vi "Main.vi"(8 "error in":errorcluster, 11 "Save Data in":refnum<class "Save Data.lvclass">) -> (0 "error out":errorcluster, 3 "Save Data out":refnum<class "Save Data.lvclass">)   [LabVIEW 2018, in "Save Data.lvclass"]
doc: "The Queued Message Handler of a Worker."
uses:
  Save Data.lvclass
  Save Data.lvclass/Save Data.ctl
  Aging View/Datas.ctl
  <vilib>/drjdpowell/SQLite Library/SQL Connection/Open (path).vi
  <vilib>/drjdpowell/SQLite Library/SQL Connection/Open (string).vi
  <vilib>/AdvancedString/Path To Command Line String.vi
  <vilib>/drjdpowell/SQLite Library/SQL Connection/Execute SQL (No results).vi
  <vilib>/drjdpowell/SQLite Library/SQL Connection/Connection.lvclass
  Initialization Data.ctl
  Aging View/Aging View.lvclass
  <vilib>/drjdpowell/SQLite Library/SQLite.lvlib
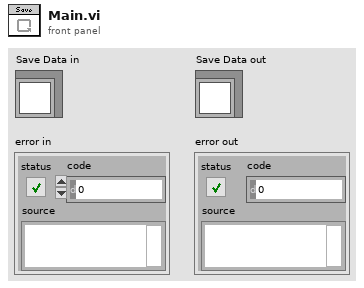
[diagram p1: front panel]
types:
  T1 = typedef "Save Data.lvclass/Initialization Data.ctl" = cluster{"MainPanel":refnum<vi>}
  T2 = typedef "Aging View.lvclass/Datas.ctl" = cluster{"Volts":dbl[], "Currents":dbl[], "Temps":dbl[]}
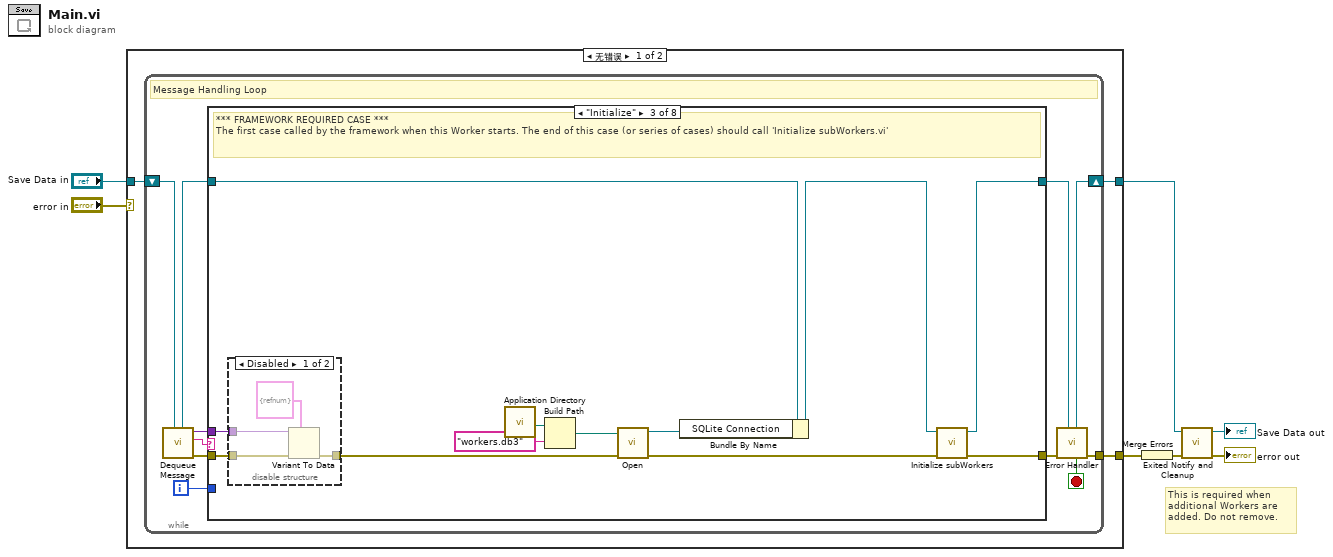
[diagram p0: block diagram]
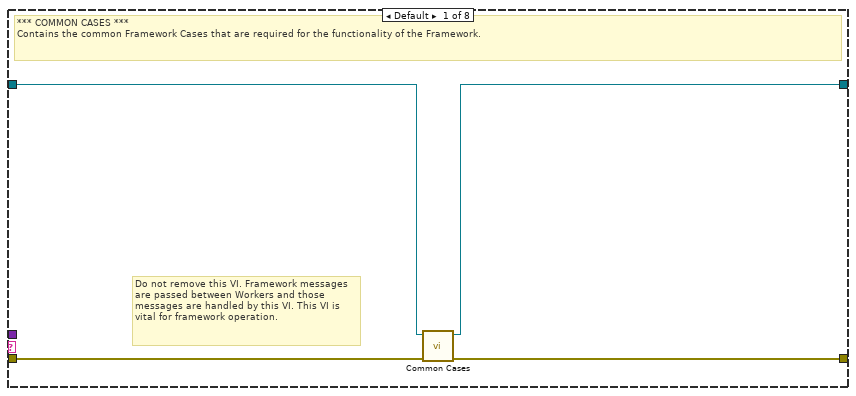
[diagram p2: hidden frame]
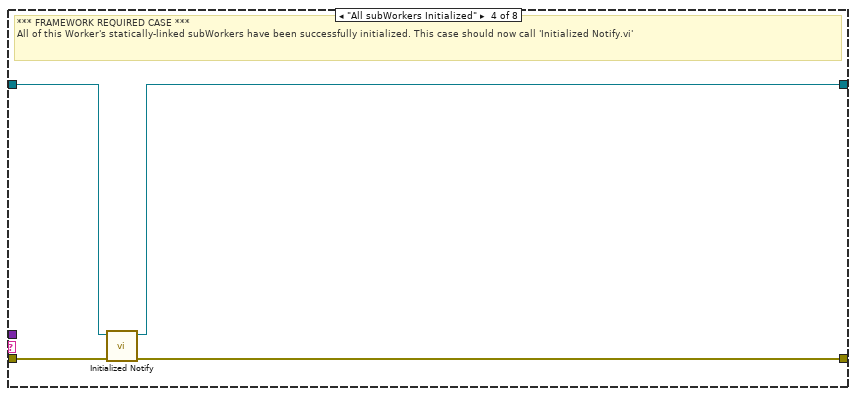
[diagram p5: hidden frame]
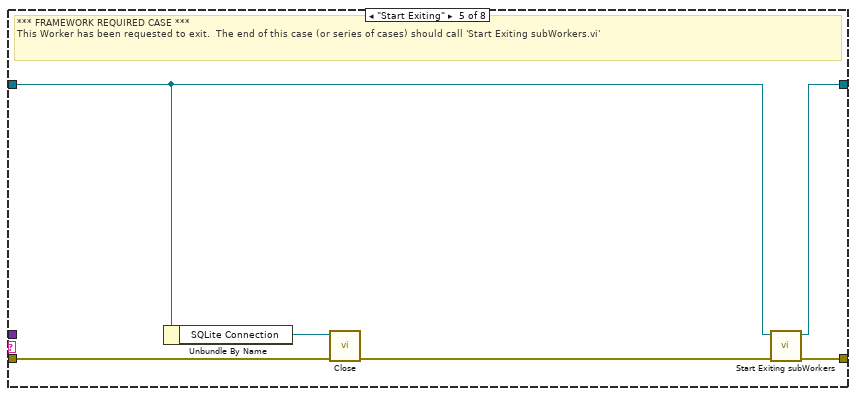
[diagram p6: hidden frame]
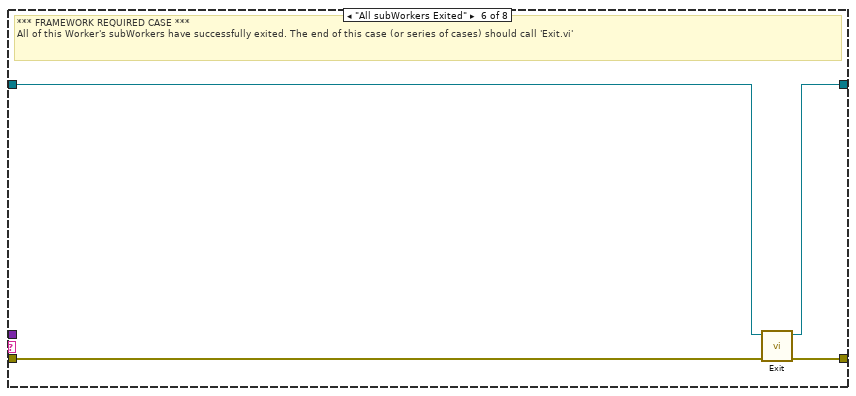
[diagram p7: hidden frame]
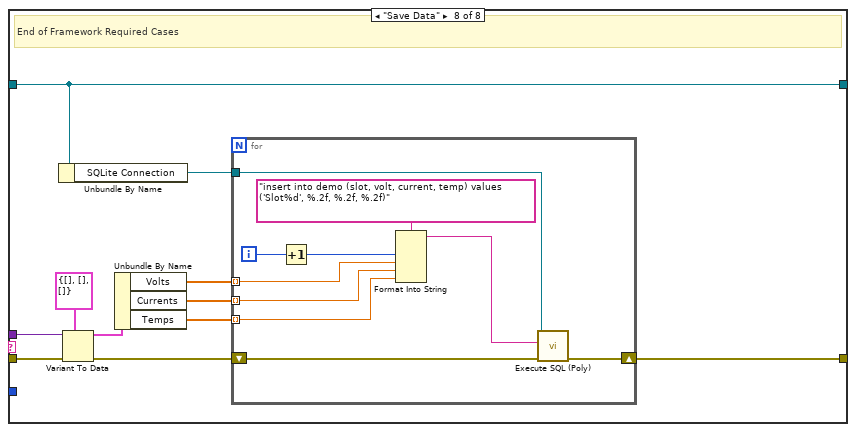
[diagram p9: hidden frame]
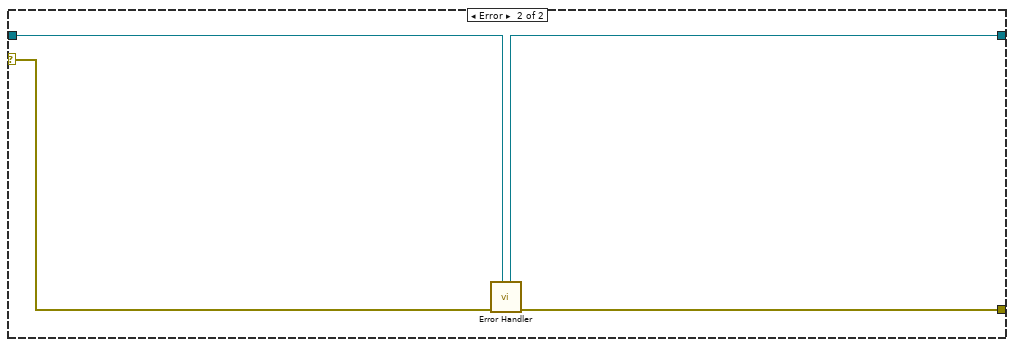
[diagram p10: hidden frame]
diagram:
  # "This is required when additional Workers are added. Do not remove."
  n1 = case shown="无错误" "error in" {
    tunnel: "Save Data in" -> [w8 w83]
    tunnel: [w10 w84] -> w6
    tunnel: [w9 w82] -> w7
    selector: "error in" -> [_ w85]
    frame No Error {
      n2 = while {
        shift-right: [w19] -> w9
        shift-left: w8 -> [w21]
        tunnel: [w20] -> w10
        i -> [w11]
        stop <- w12 stop-if-true
        # "Message Handling Loop"
        n3 = call-dynamic "Dequeue Message.vi"("Worker"=w21) -> ("error out"=w18:errorcluster, "Case out"=w13:string, "Data out"=w14:variant, "Worker out"=w16:refnum<class "Save Data.lvclass">)  [unwired: 6 in, 1 out]
        n4 = case "Worker MHL Case Structure (DO NOT CHANGE LABEL NAME)" shown="\"Initialize\"" w13 {
          tunnel: w18 -> [w25 w26 w37 w48 w52 w58 w59 w71]
          tunnel: [w24 w26 w39 w47 w54 w57 w59 w66] -> w17
          tunnel: w16 -> [w23 w27 w36 w46 w50 w56 w60 w65]
          tunnel: [w22 w27 w38 w45 w53 w55 w60 w65] -> w15
          tunnel: w14 -> [_ _ w35 _ _ _ _ w70]
          tunnel: w11 -> [_ _ _ _ _ _ _ _]
          frame Default {
            # "Do not remove this VI. Framework messages are passed between Workers and those messages are handled by this VI. This VI is vital for framework operation."
            # "*** COMMON CASES ***\nContains the common Framework Cases that are required for the functionality of the Framework."
            n5 = call-dynamic "Common Cases.vi"("error in"=w25, "Worker in"=w23) -> ("error out"=w24:errorcluster, "Worker out"=w22:refnum<class "Save Data.lvclass">)  [unwired: 8 in]
          }
          frame "------ FRAMEWORK REQUIRED CASES ------" {
            # "Start of Framework Required Cases"
          }
          frame "Initialize" {
            # "*** FRAMEWORK REQUIRED CASE ***\nThe first case called by the framework when this Worker starts. The end of this case (or series of cases) should call 'Initialize subWorkers.vi'"
            n6 = disable-structure shown="Disabled" {
              disable-tunnel: w37 -> [w43 w44]
              disable-tunnel: [w42 w44] -> w34
              disable-tunnel: w35 -> [w40 _]
              frame Disabled {
                n7 = Variant To Data(error in=w43, type=T1 {"MainPanel"=refnum} ("Cluster"), Variant=w40) -> (error out=w42:errorcluster)  [unwired: 1 out]
              }
              frame Enabled {
              }
            }
            n8 = call <vilib>:"Application Directory.vi"() -> ("Application Directory"=w33:path)
            n9 = Build Path(base path=w33, name or relative path="workers.db3") -> (appended path=w31:path)
            n10 = call-poly <vilib>:"Open.vi"("error in (no error)"=w34, "db file"=w31) -> ("error out"=w28:errorcluster, "SQLite Connection"=w29:refnum<class "Connection.lvclass">)  [unwired: 8 in]
            n11 = Bundle By Name(cluster=w36, "SQLite Connection"=w29) -> (w30:refnum<class "Save Data.lvclass">)
            n12 = call-dynamic "Initialize subWorkers.vi"("error in"=w28, "Worker"=w30) -> ("error out"=w39:errorcluster, "dup Worker out"=w38:refnum<class "Save Data.lvclass">)  [unwired: 8 in]
          }
          frame "All subWorkers Initialized" {
            # "*** FRAMEWORK REQUIRED CASE ***\nAll of this Worker's statically-linked subWorkers have been successfully initialized. This case should now call 'Initialized Notify.vi'"
            n13 = call-dynamic "Initialized Notify.vi"("error in"=w48, "Worker"=w46) -> ("error out"=w47:errorcluster, "dup Worker out"=w45:refnum<class "Save Data.lvclass">)  [unwired: 8 in]
          }
          frame "Start Exiting" {
            # "*** FRAMEWORK REQUIRED CASE ***\nThis Worker has been requested to exit.  The end of this case (or series of cases) should call 'Start Exiting subWorkers.vi'"
            n14 = Unbundle By Name(w50) -> ("SQLite Connection"=w49:refnum<class "Connection.lvclass">)
            n15 = call-dynamic "Close.vi"("error in (no error)"=w52, "SQLite Connection in"=w49) -> ("error out"=w51:errorcluster)  [unwired: 9 in]
            n16 = call-dynamic "Start Exiting subWorkers.vi"("error_in"=w51, "Worker"=w50) -> ("error out"=w54:errorcluster, "dup Worker out"=w53:refnum<class "Save Data.lvclass">)  [unwired: 8 in]
          }
          frame "All subWorkers Exited" {
            # "*** FRAMEWORK REQUIRED CASE ***\nAll of this Worker's subWorkers have successfully exited. The end of this case (or series of cases) should call 'Exit.vi'"
            n17 = call-dynamic "Exit.vi"("error_in"=w58, "Worker"=w56) -> ("error out"=w57:errorcluster, "dup Worker out"=w55:refnum<class "Save Data.lvclass">)  [unwired: 8 in]
          }
          frame "-----------------------------------------------" {
            # "End of Framework Required Cases"
          }
          frame "Save Data" {
            # "End of Framework Required Cases"
            n18 = Unbundle By Name(w65) -> ("SQLite Connection"=w64:refnum<class "Connection.lvclass">)
            n19 = Variant To Data(error in=w71, type=T2 {"Volts"=[], "Currents"=[], "Temps"=[]} ("Datas"), Variant=w70) -> (data=w68:T2, error out=w67:errorcluster)
            n20 = Unbundle By Name(w68) -> ("Volts"=w63:dbl[], "Currents"=w62:dbl[], "Temps"=w61:dbl[])
            n21 = for {
              shift-right: [w80] -> w66
              shift-left: w67 -> [w81]
              tunnel: w64 -> [w79]
              tunnel: w63 -> [w75] mode=indexing
              tunnel: w62 -> [w74] mode=indexing
              tunnel: w61 -> [w73] mode=indexing
              i -> [w77]
              n22 = Increment(x=w77) -> (x+1=w76:i32)
              n23 = Format Into String(format string="insert into demo (slot, volt, current, temp) values ('Slot%d', %.2f, %.2f, %.2f)", w76, w75, w74, w73) -> (resulting string=w72:string)  [unwired: 2 in, 1 out]
              n24 = call-poly <vilib>:"Execute SQL (Poly).vi"("error in (no error)"=w81, "SQL"=w72, "SQLite Connection in"=w79) -> ("error out"=w80:errorcluster)  [unwired: 7 in, 1 out]
            }
          }
        }
        n25 = call-dynamic "Error Handler.vi"("Worker"=w15, "error_in"=w17) -> ("error out"=w20:errorcluster, "Stop Loop"=w12:bool, "Worker out"=w19:refnum<class "Save Data.lvclass">)  [unwired: 7 in]
      }
    }
    frame Error {
      n26 = call-dynamic "Error Handler.vi"("Worker"=w83, "error_in"=w85) -> ("error out"=w84:errorcluster, "Worker out"=w82:refnum<class "Save Data.lvclass">)  [unwired: 7 in, 1 out]
    }
  }
  n27 = Merge Errors(w6) -> (w3:errorcluster)
  n28 = call-dynamic "Exited Notify and Cleanup.vi"("error_in"=w3, "Worker"=w7) -> ("error out"=→"error out":errorcluster, "dup Worker out"=→"Save Data out":refnum<class "Save Data.lvclass">)  [unwired: 8 in]
